vi "Read Experiment Path.vi"(8 "error in (no error)":errorcluster, 11 "AFM Control":refnum<class "AFM Control.lvclass">) -> (0 "error out":errorcluster, 2 "Experiment Path":path, 3 "AFM Control out":refnum<class "AFM Control.lvclass">)   [LabVIEW 2016, in "AFM Control.lvclass"]
uses:
  AFM Control.lvclass
  AFM Control.lvclass/AFM Control.ctl
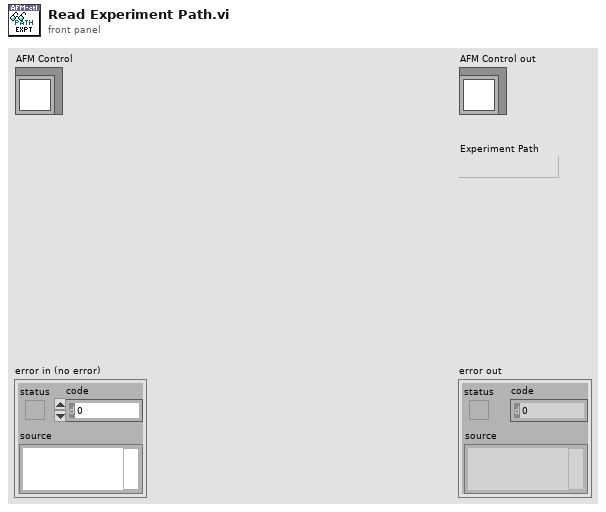
[diagram p1: front panel]
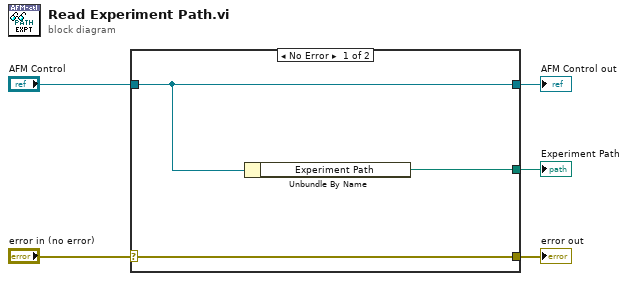
[diagram p0: block diagram]
diagram:
  n1 = case shown="No Error" "error in (no error)" {
    selector: "error in (no error)" -> [w8 w9]
    tunnel: [w8 w9] -> w4
    tunnel: [w7 w10] -> w2
    tunnel: "AFM Control" -> [w7 w10]
    tunnel: [w6 _] -> w1
    frame No Error {
      n2 = Unbundle By Name(w7) -> ("Experiment Path"=w6:path)
    }
    frame Error {
    }
  }
  "error out" <- w4
  "AFM Control out" <- w2
  "Experiment Path" <- w1
